vi "Lamp.vi"() -> (0 "error out":errorcluster)   [LabVIEW 2016]
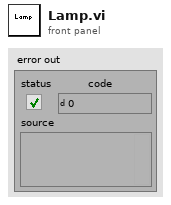
[diagram p1: front panel]
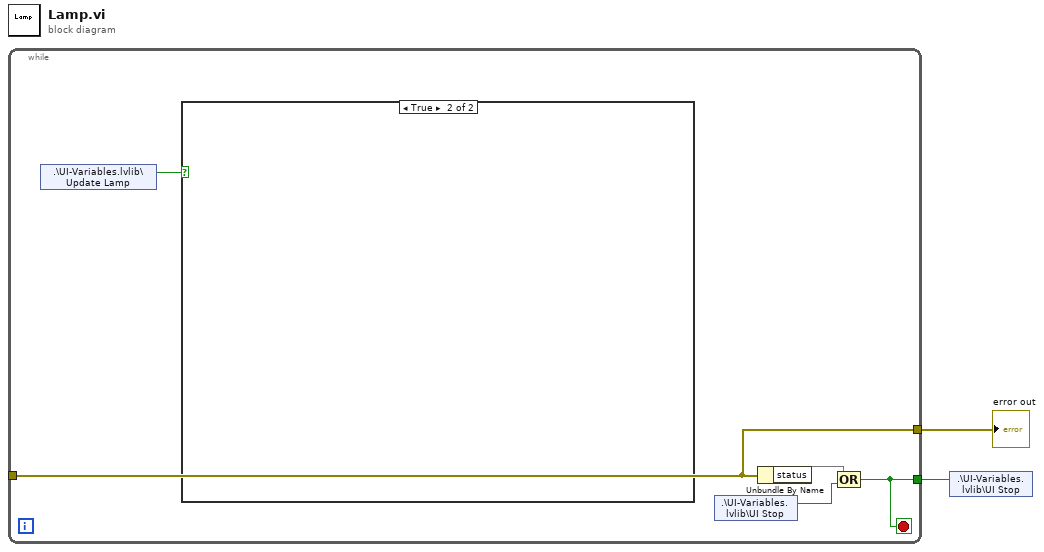
[diagram p0: block diagram]
diagram:
  n1 = while {
    tunnel: [w5] -> w1
    tunnel: [w6] -> w3
    tunnel: [w5] -> w2
    stop <- w6 stop-if-true
    n2 = shared-variable ".\\UI-Variables.lvlib\\Update Lamp"() -> (w4:bool)  [unwired: 1 in, 1 out]
    n3 = case shown="True" w4 {
      frame False {
      }
      frame True {
      }
    }
    n4 = shared-variable ".\\UI-Variables.lvlib\\UI Stop"() -> (w8:bool)  [unwired: 1 in, 1 out]
    n5 = Unbundle By Name(w5) -> ("status"=w7)
    n6 = Compound Arithmetic op=OR(w7, w8) -> (w6:bool)
  }
  "error out" <- w2
  n7 = shared-variable ".\\UI-Variables.lvlib\\UI Stop"(w3) -> ()  [unwired: 1 in, 1 out]
